vi "AM Cross Compare Temp Data.vi"(7 "Temp Length":i32[](array[numeric]), 11 "All Data Cluster":cluster{"Splitted Data":dbl[], dbl[]}[](array[cluster])) -> (1 "Small SG Vector":dbl[](array[numeric]), 2 "Cross Index":i32, 3 "Longest SG Vector":dbl[](array[numeric]), 4 "Longest Temp Vector":dbl[](array[numeric]))   [LabVIEW 2020, in "Test Driver.lvlib"]
uses:
  Test Driver.lvlib
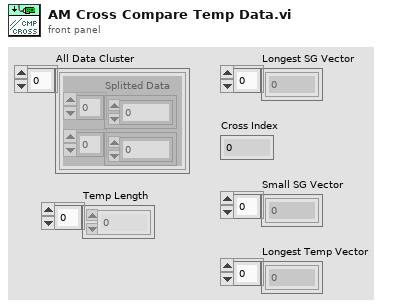
[diagram p1: front panel]
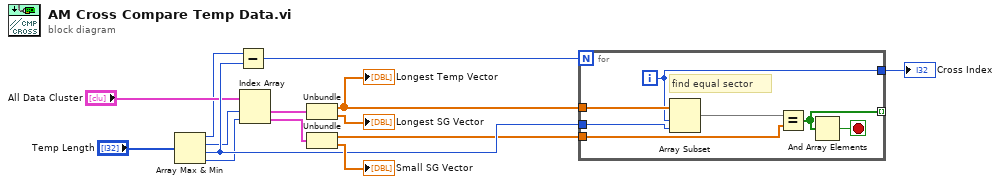
[diagram p0: block diagram]
diagram:
  n1 = Array Max & Min(array="Temp Length") -> (max value=w2:i32, max index (indices)=w5:i32, min value=w10:i32, min index (indices)=w6:i32)
  n2 = Subtract(x=w2, y=w10) -> (x-y=w3:i32)
  n3 = Index Array(array="All Data Cluster", index #1=w5, index #2=w6) -> (element #1=w7:cluster{"Splitted Data":dbl[], dbl[]}, element #2=w8:cluster{"Splitted Data":dbl[], dbl[]})
  n4 = Unbundle(w7) -> ("Splitted Data"=w14:dbl[], →"Longest SG Vector":dbl[])
  "Longest Temp Vector" <- w14
  n5 = Unbundle(w8) -> ("Splitted Data"=w9:dbl[], →"Small SG Vector":dbl[])
  n6 = for {
    N: w3 -> [_]
    tunnel: w14 -> [w21]
    tunnel: w9 -> [w18]
    tunnel: w10 -> [w20]
    tunnel: [w17] -> _ mode=indexing
    tunnel: [w15] -> w12
    i -> [w15]
    stop <- w16 stop-if-true
    # "find equal sector"
    n7 = Array Subset(array=w21, index=w15, length=w20) -> (w19:dbl[])
    n8 = Equal?(x=w19, y=w18) -> (x = y?=w17:bool[])
    n9 = And Array Elements(Boolean array=w17) -> (logical AND=w16:bool)
  }
  "Cross Index" <- w12
